vi "Master Method Version.vi"(7 "Config":T1, 9 "error in (no error)":errorcluster, 11 "Master Method version":i32) -> (1 "error out":errorcluster, 2 "Current Master Method Version":i32, 3 "Master Method Version":i32, 5 "found?":bool)   [LabVIEW 2012]
uses:
  ReadWrite.ctl
  <vilib>/Utility/config.llb/Read Key (I32).vi
  <vilib>/Utility/config.llb/Write Key (I32).vi
  Design Server.lvlib
  <vilib>/Utility/config.llb/NI_LVConfig.lvlib
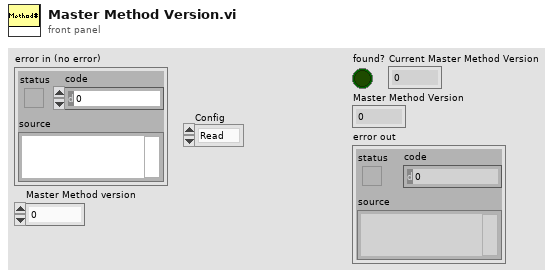
[diagram p1: front panel]
types:
  T1 = typedef "ReadWrite.ctl" = enum16{"Read", "Write"}
  T2 = typedef "NI_LVConfig.lvlib/Config Data RefNum.ctl" = refnum<k1>
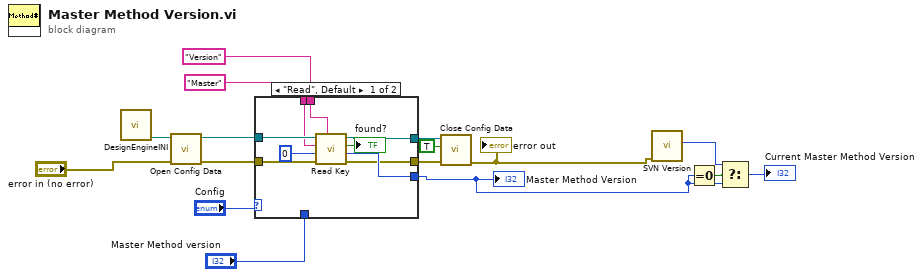
[diagram p0: block diagram]
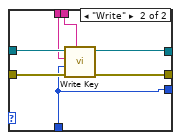
[diagram p2: hidden frame]
diagram:
  n1 = call "DesignEngineINI.vi"() -> ("Ini file path"=w15:path)  [unwired: 6 in, 1 out]
  n2 = call <vilib>:"Open Config Data.vi"("error in (no error)"="error in (no error)", "configuration file path"=w15) -> ("error out"=w16:errorcluster, "refnum"=w14:T2)  [unwired: 7 in, 1 out]
  n3 = case shown="\"Read\", Default" "Config" {
    tunnel: w16 -> [w25 w28]
    tunnel: w14 -> [w24 w32]
    tunnel: [w21 w26] -> w2
    tunnel: "Master" ("section") -> [w20 w29]
    tunnel: "Version" ("section") -> [w19 w30]
    tunnel: [w18 w31] -> w10
    tunnel: [w17 w27] -> w9
    tunnel: "Master Method version" -> [_ w26]
    frame "Read", Default {
      n4 = call-poly <vilib>:"Read Key.vi"("section"=w19, "error in (no error)"=w25, "default value"=0, "key"=w20, "refnum"=w24) -> ("error out"=w17:errorcluster, "value"=w21:i32, "found?"=→"found?":bool, "refnum out"=w18:T2)  [unwired: 3 in]
    }
    frame "Write" {
      n5 = call-poly <vilib>:"Write Key.vi"("section"=w30, "error in (no error)"=w28, "value"=w26, "key"=w29, "refnum"=w32) -> ("error out"=w27:errorcluster, "refnum out"=w31:T2)  [unwired: 4 in, 1 out]
    }
  }
  "Master Method Version" <- w2
  n6 = call <vilib>:"Close Config Data.vi"("error in (no error)"=w9, "write file if changed (T)"=TRUE, "refnum"=w10) -> ("error out"=w3:errorcluster)  [unwired: 7 in, 1 out]
  "error out" <- w3
  n7 = call "SVN Version.vi"("error in (no error)"=w3) -> ("Revision"=w4:i32)  [unwired: 7 in, 3 out]
  n8 = Equal To 0?(x=w2) -> (x = 0?=w5:bool)
  n9 = Select(t=w4, s=w5, f=w2) -> (s? t:f=→"Current Master Method Version":i32)
